vi "Convert Actual Column to Selected Message Log Column.vi"(10 "Visible ML Columns":bool[](array[boolean]), 11 "Actual Column":i32=1) -> (3 "Selected Column":i32)   [LabVIEW 2017, in "Message Log.lvclass"]
uses:
  Message Log.lvclass
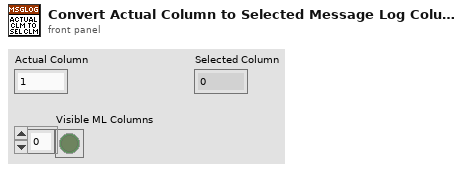
[diagram p1: front panel]
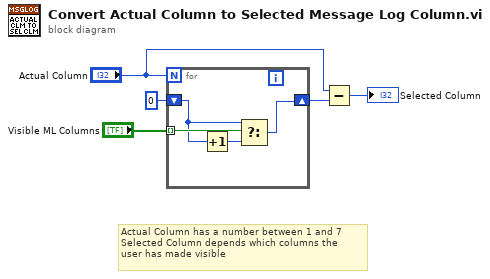
[diagram p0: block diagram]
diagram:
  # "Actual Column has a number between 1 and 7\nSelected Column depends which columns the \nuser has made visible"
  n1 = for {
    N: "Actual Column" -> [_]
    tunnel: "Visible ML Columns" -> [w9] mode=indexing
    shift-right: [w7] -> w3
    shift-left: 0 -> [w8]
    n2 = Increment(x=w8) -> (x+1=w6:i32)
    n3 = Select(t=w8, s=w9, f=w6) -> (s? t:f=w7:i32)
  }
  n4 = Subtract(x="Actual Column", y=w3) -> (x-y=→"Selected Column":i32)
